vi "Setup UI.vi"(8 "error in":errorcluster, 10 "Set UI to input? (F)":bool, 11 "Continuous.lvclass":refnum<class "Continuous.lvclass">) -> (0 "error out":errorcluster, 3 "Continuous.lvclass out":refnum<class "Continuous.lvclass">)   [LabVIEW 2017, in "Continuous.lvclass"]
uses:
  Continuous.lvclass
  Continuous.lvclass/Continuous.ctl
panel:
  out "Suggested dwell time per point":dbl[unit]
  in  "specifyrate":bool=TRUE
  in  "Total Time for Scan":dbl[unit]
  in  "Sweep Rate":dbl[unit] min=0.0 max=0.016666666666666666
  in  "Temperature":dbl
  # "specify by sweep rate"
  # "specify by total time"
  # "1"
  # "2"
  # "Continuous B Field Scan"
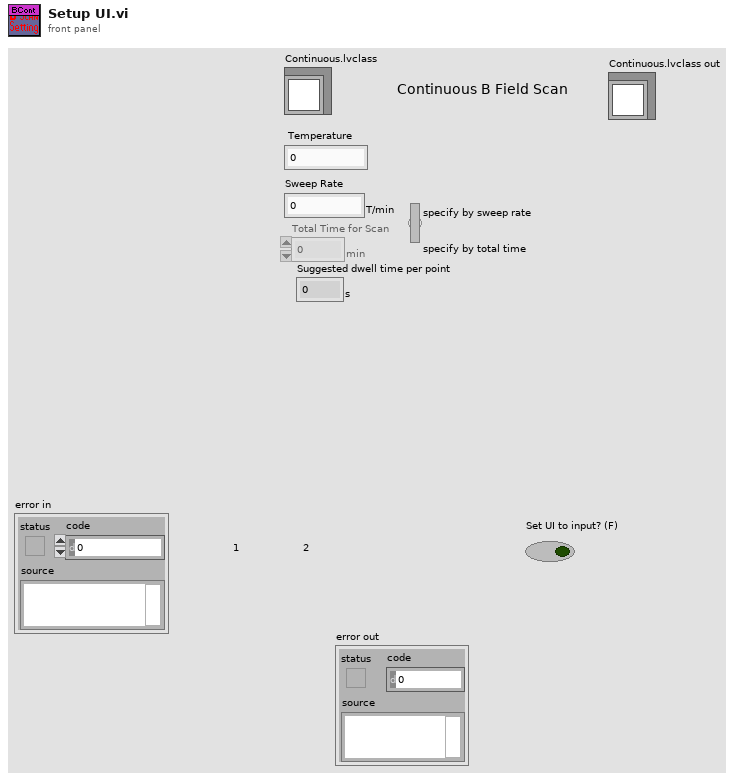
[diagram p1: front panel]
types:
  T1 = typedef "Scanner.lvclass/Range.ctl" = cluster{"xi":dbl, "xf":dbl, "dx":dbl, "Return to...?":bool, "Return to":dbl}
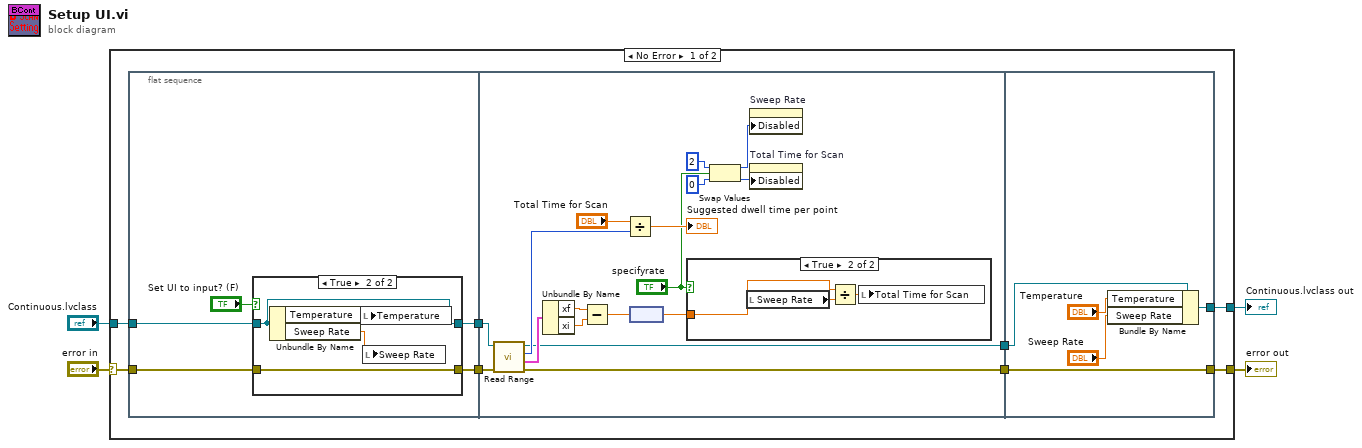
[diagram p0: block diagram]
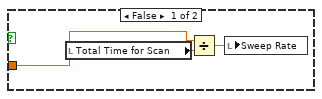
[diagram p3: hidden frame]
diagram:
  n1 = case shown="No Error" "error in" {
    selector: "error in" -> [w11 w52]
    tunnel: [w12 w52] -> w2
    tunnel: [w9 w53] -> w3
    tunnel: "Continuous.lvclass" -> [w10 w53]
    frame No Error {
      n2 = flat-sequence {
        tunnel: [w17] -> w8
        tunnel: w11 -> [w16]
        tunnel: [w15] -> w6
        tunnel: w10 -> [w14]
        tunnel: w8 -> [w27]
        tunnel: [w24] -> w7
        tunnel: w6 -> [w26]
        tunnel: [w25] -> w5
        tunnel: w7 -> [w47]
        tunnel: w5 -> [w48]
        tunnel: [w47] -> w12
        tunnel: [w49] -> w9
        frame #0 {
          n3 = case shown="True" "Set UI to input? (F)" {
            tunnel: [w19 w20] -> w17
            tunnel: w16 -> [w19 w20]
            tunnel: [w18 w23] -> w15
            tunnel: w14 -> [w18 w23]
            frame False {
            }
            frame True {
              n4 = Unbundle By Name(w23) -> ("Temperature"=w22:dbl, "Sweep Rate"=w21:dbl[unit])
              n5 = local write "Temperature"(w22) -> ()
              n6 = local write "Sweep Rate"(w21) -> ()
            }
          }
        }
        frame #1 {
          n7 = call-dynamic "Read Range.vi"("error in (no error)"=w27, "Scanner.lvclass in"=w26) -> ("error out"=w24:errorcluster, "Range"=w33:T1, "# Points"=w39:u32, "Scanner.lvclass out"=w25:refnum<class "Continuous.lvclass">)  [unwired: 6 out]
          n8 = Unbundle By Name(w33) -> ("xf"=w34:dbl, "xi"=w35:dbl)
          n9 = Subtract(x=w34, y=w35) -> (x-y=w36:dbl)
          n10 = Divide(x="Total Time for Scan", y=w39) -> (x/y=→"Suggested dwell time per point":dbl[unit])
          n11 = node(w36) -> (w37:dbl[unit])
          n12 = case shown="True" "specifyrate" {
            tunnel: w37 -> [w42 w44]
            frame False {
              n13 = local read "Total Time for Scan"() -> (w41:dbl[unit])
              n14 = Divide(x=w42, y=w41) -> (x/y=w43:dbl[unit])
              n15 = local write "Sweep Rate"(w43) -> ()
            }
            frame True {
              n16 = local read "Sweep Rate"() -> (w46:dbl[unit])
              n17 = Divide(x=w44, y=w46) -> (x/y=w45:dbl[unit])
              n18 = local write "Total Time for Scan"(w45) -> ()
            }
          }
          n19 = Swap Values(12:2 ("y"), 13:"specifyrate", 14:0 ("x")) -> (1:w28:i32, 3:w29:i32)
          n20 = property on="Sweep Rate" class="DigNum (strict)"("Disabled"=w28) -> ()  [unwired: 2 in, 2 out]
          n21 = property on="Total Time for Scan" class="DigNum (strict)"("Disabled"=w29) -> ()  [unwired: 2 in, 2 out]
        }
        frame #2 {
          n22 = Bundle By Name(cluster=w48, "Temperature"="Temperature", "Sweep Rate"="Sweep Rate") -> (w49:refnum<class "Continuous.lvclass">)
        }
      }
    }
    frame Error {
    }
  }
  "Continuous.lvclass out" <- w3
  "error out" <- w2
